vi "CRYProject Tree Mouse Check.vi"(10 "Coords In":T1, 11 "Tree Reference In":refnum<vi>) -> (2 "Clicked String Out":string, 3 "Tree Reference Out":refnum<vi>)   [LabVIEW 2013]
uses:
  <vilib>/Utility/miscctls.llb/LVPoint32TypeDef.ctl
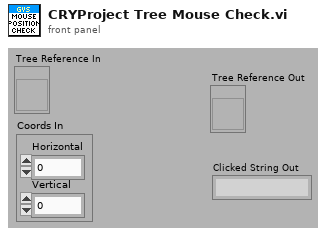
[diagram p1: front panel]
types:
  T1 = typedef "LVPoint32TypeDef.ctl" = cluster{"Horizontal":i32, "Vertical":i32}
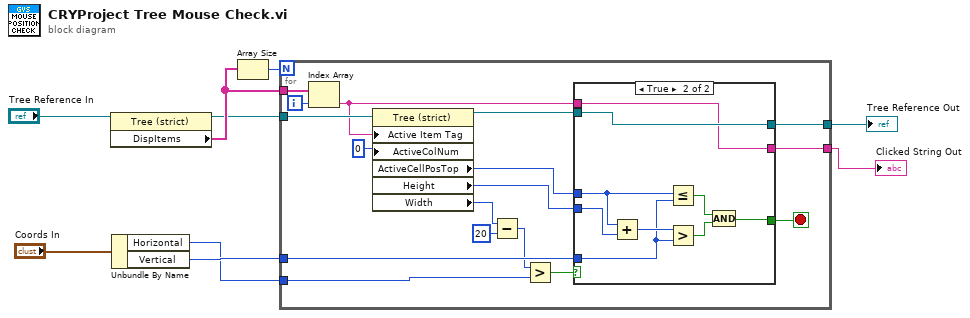
[diagram p0: block diagram]
diagram:
  n1 = property class="Tree (strict)"(reference="Tree Reference In") -> (reference out=w6:refnum<vi>, "DispItems"=w7:string[])  [unwired: 1 in, 1 out]
  n2 = Unbundle By Name("Coords In") -> ("Horizontal"=w4:i32, "Vertical"=w5:i32)
  n3 = Array Size(array=w7) -> (size(s)=w3:i32)
  n4 = for {
    N: w3 -> [_]
    tunnel: w6 -> [w26]
    tunnel: w5 -> [w20]
    tunnel: w7 -> [w24]
    tunnel: w4 -> [w16]
    tunnel: [w12] -> w2
    tunnel: [w10] -> w1
    i -> [w25]
    stop <- w13 stop-if-true
    n5 = Index Array(array=w24, index=w25) -> (element=w23:string)
    n6 = property class="Tree (strict)"(reference=w26, "Active Item Tag"=w23, "ActiveColNum"=0 ("Active Cell:Active Column Number")) -> (reference out=w19:refnum<vi>, "ActiveCellPosTop"=w22:i32, "Height"=w21:i32, "Width"=w18:i32)  [unwired: 1 in, 1 out]
    n7 = Subtract(x=w18, y=20) -> (x-y=w17:i32)
    n8 = Greater?(x=w17, y=w16) -> (0:w15:bool)
    n9 = case shown="True" w15 {
      selector: w15 -> [w29 _]
      tunnel: w23 -> [w27 w30]
      tunnel: w22 -> [_ w36]
      tunnel: w21 -> [_ w34]
      tunnel: w20 -> [_ w33]
      tunnel: w19 -> [w28 w31]
      tunnel: [w29 w32] -> w13
      tunnel: [w28 w31] -> w12
      tunnel: [w27 w30] -> w10
      frame False {
      }
      frame True {
        n10 = Add(x=w36, y=w34) -> (x+y=w35:i32)
        n11 = Less Or Equal?(x=w36, y=w33) -> (x <= y?=w37:bool)
        n12 = Greater?(x=w35, y=w33) -> (0:w38:bool)
        n13 = Compound Arithmetic op=AND(w37, w38) -> (w32:bool)
      }
    }
  }
  "Tree Reference Out" <- w2
  "Clicked String Out" <- w1
